vi "test Parse Timestamp Array2.vi"(11 "Test Case In":refnum<class "Test Named Fields Parser.lvclass">) -> (0 "error out":errorcluster, 3 "Test Case Out":refnum<class "Test Named Fields Parser.lvclass">)   [LabVIEW 2024, in "Test Named Fields Parser.lvclass"]
uses:
  Test Named Fields Parser.lvclass
  C:/Program Files/National Instruments/LabVIEW 2025/vi.lib/Astemes/LUnit/Test Case.lvclass
  CSV Parser/Named Fields Parser/Named Fields Parser.lvclass
  <vilib>/Astemes/LUnit/Test Case.lvclass/Test Case.ctl
  Test Named Fields Parser.lvclass/Test Named Fields Parser.ctl
  <vilib>/Astemes/LUnit/Test Case.lvclass
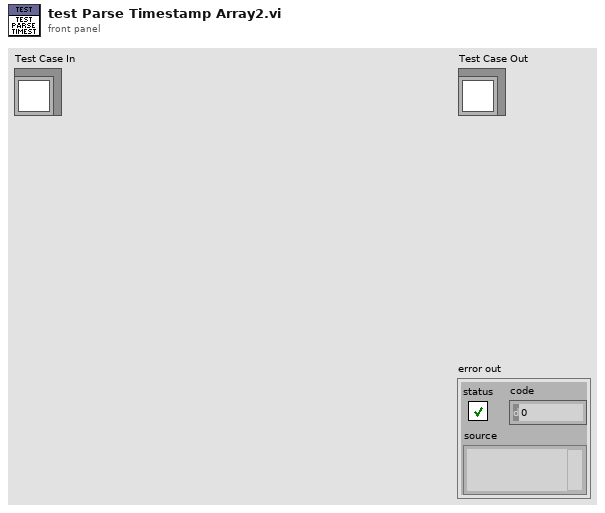
[diagram p1: front panel]
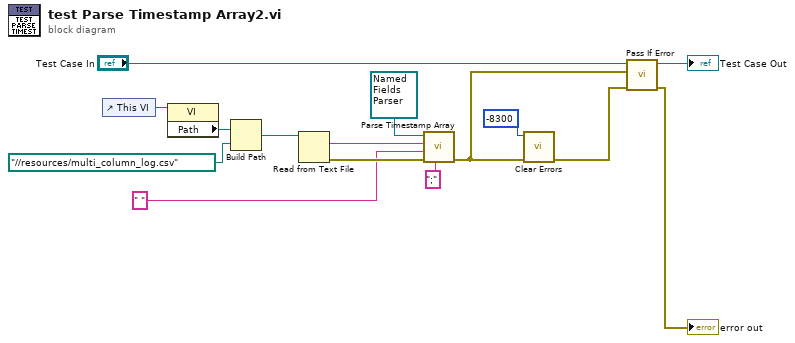
[diagram p0: block diagram]
diagram:
  n1 = control-ref of="This VI"() -> (w12:refnum<vi>)
  n2 = property class="VI"(reference=w12) -> ("Path"=w11:path)  [unwired: 1 in, 2 out]
  n3 = Build Path(base path=w11, name or relative path=path "../../resources/multi_column_log.csv" ("file (use dialog)")) -> (appended path=w10:path)
  n4 = Read from Text File(file (use dialog)=w10) -> (text=w9:string, error out=w8:errorcluster)  [unwired: 3 in, 2 out]
  n5 = call-dynamic "Parse Timestamp Array.vi"("Seperator"=";", "error in"=w8, "Input"=" " ("Input <JSON>"), "csv string"=w9, "Named Columns Parser in"=refnum<class "Named Fields Parser.lvclass"> refnum) -> ("error out"=w3:errorcluster)  [unwired: 4 in, 2 out]
  n6 = call <vilib>:"Clear Errors.vi"("error in (no error)"=w3, "specific error code to clear (0: all)"=-8300) -> ("error out"=w2:errorcluster)  [unwired: 4 in, 1 out]
  n7 = call <vilib>:"Pass If Error.vi"("error in (no error)"=w2, "Assert error"=w3, "LUnit Test Case In"="Test Case In") -> ("error out"=→"error out":errorcluster, "LUnit Test Case Out"=→"Test Case Out":refnum<class "Test Named Fields Parser.lvclass">)  [unwired: 7 in]
